vi "box detector.vi"() -> ()   [LabVIEW 2026]
panel:
  in  "stop":bool
  in  "Slide":dbl(slide) scale=0.0..10.0
  out "sensor 2":bool
  out "sensor":bool
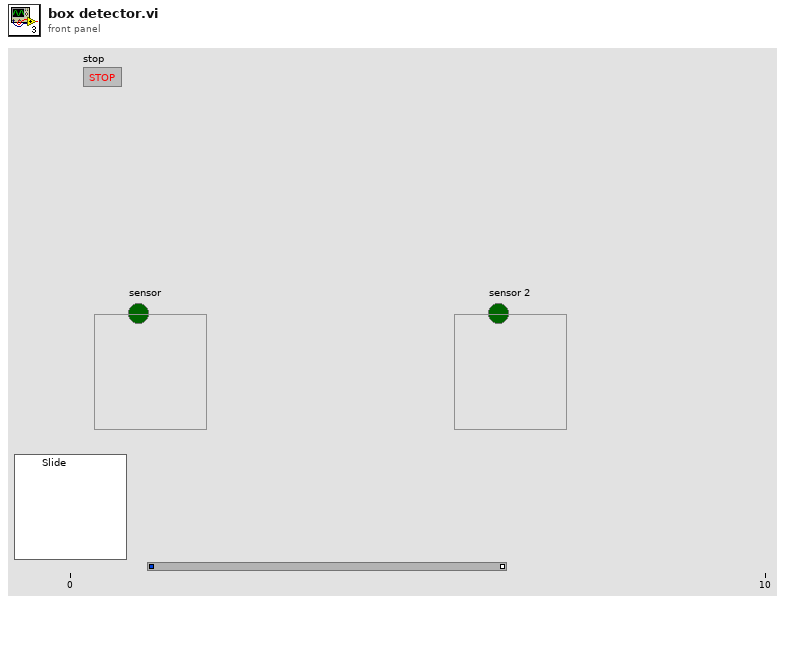
[diagram p1: front panel]
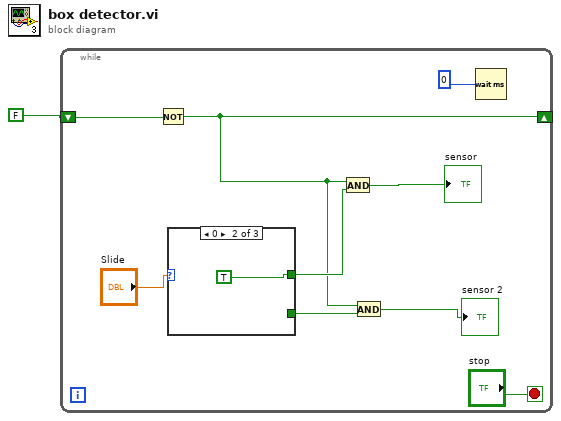
[diagram p0: block diagram]
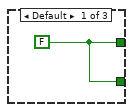
[diagram p2: hidden frame]
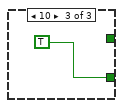
[diagram p3: hidden frame]
diagram:
  n1 = while {
    shift-right: [w6] -> _
    shift-left: FALSE -> [w10]
    stop <- "stop" stop-if-true
    n2 = Not(x=w10) -> (.not. x?=w6:bool)
    n3 = case shown="0" "Slide" {
      tunnel: [w11 TRUE _] -> w7
      tunnel: [w11 _ TRUE] -> w5
      frame Default {
        w11 = FALSE
      }
      frame 0 {
      }
      frame 10 {
      }
    }
    n4 = And(x=w6, y=w7) -> (x .and. y?=→"sensor":bool)
    n5 = And(x=w6, y=w5) -> (x .and. y?=→"sensor 2":bool)
    n6 = Wait (ms)(milliseconds to wait=u32 0) -> ()  [unwired: 1 out]
  }
